vi "Format Last Update.vi"(11 "Last Update":dbl) -> (3 "Last Update String":string)   [LabVIEW 2020, in "PicoG-Processor.lvlib" / "WebProjectPanel.lvclass"]
uses:
  WebProjectPanel.lvclass
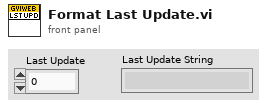
[diagram p1: front panel]
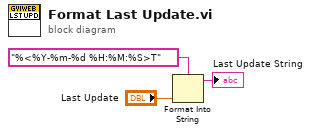
[diagram p0: block diagram]
diagram:
  n1 = Format Into String(format string="%<%Y-%m-%d %H:%M:%S>T", "Last Update") -> (resulting string=→"Last Update String":string)  [unwired: 2 in, 1 out]
